vi "InitApplication_HH.vi"(0 "file name":string, 1 "VI path":path) -> ()   [LabVIEW 2009]
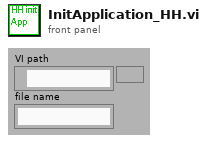
[diagram p1: front panel]
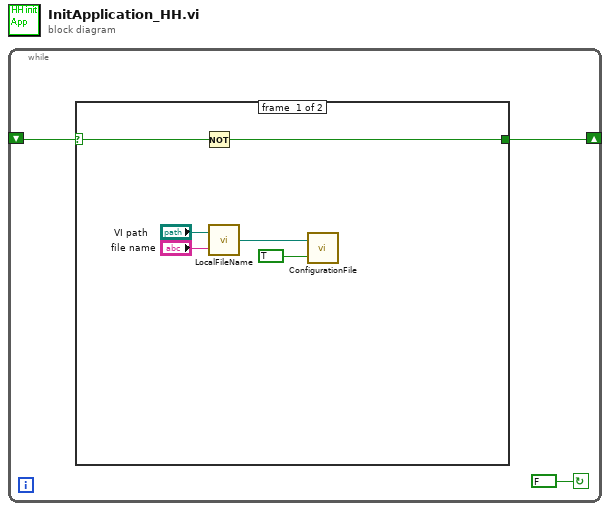
[diagram p0: block diagram]
diagram:
  n1 = while {
    shift-right: [w1] -> _
    shift-left: _ -> [w2]
    stop <- FALSE continue-if-true
    n2 = case shown="False" w2 {
      selector: w2 -> [w9 w10]
      tunnel: [w8 w10] -> w1
      frame #0 {
        n3 = Not(x=w9) -> (.not. x?=w8:bool)
        n4 = call "LocalFileName.vi"("file name"="file name", "VI path"="VI path") -> ("full path"=w6:path)
        n5 = call "ConfigurationFile.vi"("Set/Get"=TRUE, "Configuration File (input)"=w6) -> ()  [unwired: 1 out]
      }
      frame #1 {
      }
    }
  }
